vi "Is Sequential.vi"(8 "error in (no error)":errorcluster, 11 "Transfer Configuration in":refnum<class "Configuration.Transfer.lvclass">) -> (0 "error out":errorcluster, 2 "sequential offsets?":bool, 3 "Transfer Configuration out":refnum<class "Configuration.Transfer.lvclass">)   [LabVIEW 2016, in "Configuration.Transfer.lvclass"]
uses:
  Configuration.Transfer.lvclass
  Configuration.Transfer.lvclass/Configuration.Transfer.ctl
  Configuration.Channel/Configuration.Channel.lvclass/Configuration.Channel.ctl
  Configuration.Channel/Configuration.Channel.lvclass
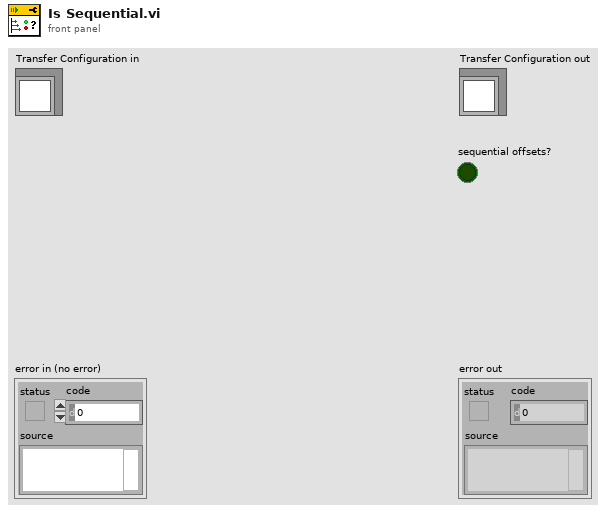
[diagram p1: front panel]
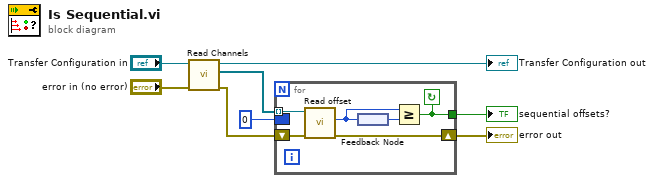
[diagram p0: block diagram]
diagram:
  n1 = call "Read Channels.vi"("error in (no error)"="error in (no error)", "Configuration.Transfer in"="Transfer Configuration in") -> ("error out"=w2:errorcluster, "Channels"=w7:refnum<class "Configuration.Channel.lvclass">[], "Configuration.Transfer out"=→"Transfer Configuration out":refnum<class "Configuration.Transfer.lvclass">)  [unwired: 7 in]
  n2 = for {
    tunnel: w7 -> [w14] mode=indexing
    border: u64 0 ("offset") -> [_]
    tunnel: [w11] -> w5
    shift-right: [w9] -> w1
    shift-left: w2 -> [w10]
    stop <- w11 continue-if-true
    n3 = call "Read offset.vi"("error in (no error)"=w10, "Configuration.Channel in"=w14) -> ("error out"=w9:errorcluster, "offset"=w13:u64)  [unwired: 7 in, 1 out]
    n4 = feedback-in #1(w13) -> ()
    n5 = feedback #1() -> (w12:u64)
    n6 = Greater Or Equal?(x=w13, y=w12) -> (x >= y?=w11:bool)
  }
  "error out" <- w1
  "sequential offsets?" <- w5
